vi "LoadDeviceList.vi"(8 "error in":errorcluster, 9 "usb/RS170":bool, 11 "path to XML document":path) -> (0 "error out":errorcluster, 1 "parse errors":string, 3 "DeviceList":T2(array[cluster]) {"Acquisition Parameters"."White level" scale=0.3..1.26 scale format="%#_2f"; "Acquisition Parameters"."Saturation" scale=0.5..1.5 scale format="%#_3f"; "Acquisition Parameters"."Contrast" scale=0.4..1.5 scale format="%#_3f"; "Acquisition Parameters"."Brightness" scale=-50.0..50.0 scale format="%#_2f"; "Correction Parameters"."Movement Type" items=["Step", "Proportionnal"]; "Target"."X Target" format="%#_5g"; "Target"."Y Target" format="%#_5g"; "Detection Parameters"."Max Intensity%" max=100 step=1})   [LabVIEW 2013]
uses:
  <vilib>/xml/Load XML File.vi
  <vilib>/xml/NI_XML.lvlib
  <resource>/objmgr/DOMUserDefRef.rc
panel:
  out "ImageServer":cluster{"IPAddress":string, "Port":i32}
  out "YCalibration":cluster{dbl, dbl}[](graph)
  out "XCalibration":cluster{dbl, dbl}[](graph)
  out "ID":i32
  out "Name":string
  out "DeviceID":T1
  out "Reference Path":path
  out "Background Path":path
  out "Acquisition Parameters":T3={"Brightness"=0.0, "Contrast"=1.0, "Saturation"=1.0, "White level"=0.7} {"White level" scale=0.3..1.26 scale format="%#_2f"; "Saturation" scale=0.5..1.5 scale format="%#_3f"; "Contrast" scale=0.4..1.5 scale format="%#_3f"; "Brightness" scale=-50.0..50.0 scale format="%#_2f"}
  out "Reverse":cluster{"Reverse X":bool, "Reverse Y":bool}
  out "Target":cluster{"X Target":sgl, "Y Target":sgl} {"X Target" format="%#_5g"; "Y Target" format="%#_5g"}
  out "Region of Interest":i32[](array[numeric])=[-1, -1, 32000, 32000]
  out "Correction Parameters":cluster{"X":sgl, "Y":sgl, "Movement Type":u16}={"X"=5.0, "Y"=5.0, "Movement Type"=0} {"Movement Type" items=["Step", "Proportionnal"]}
  out "Detection Parameters":T4 {"Max Intensity%" max=100 step=1}
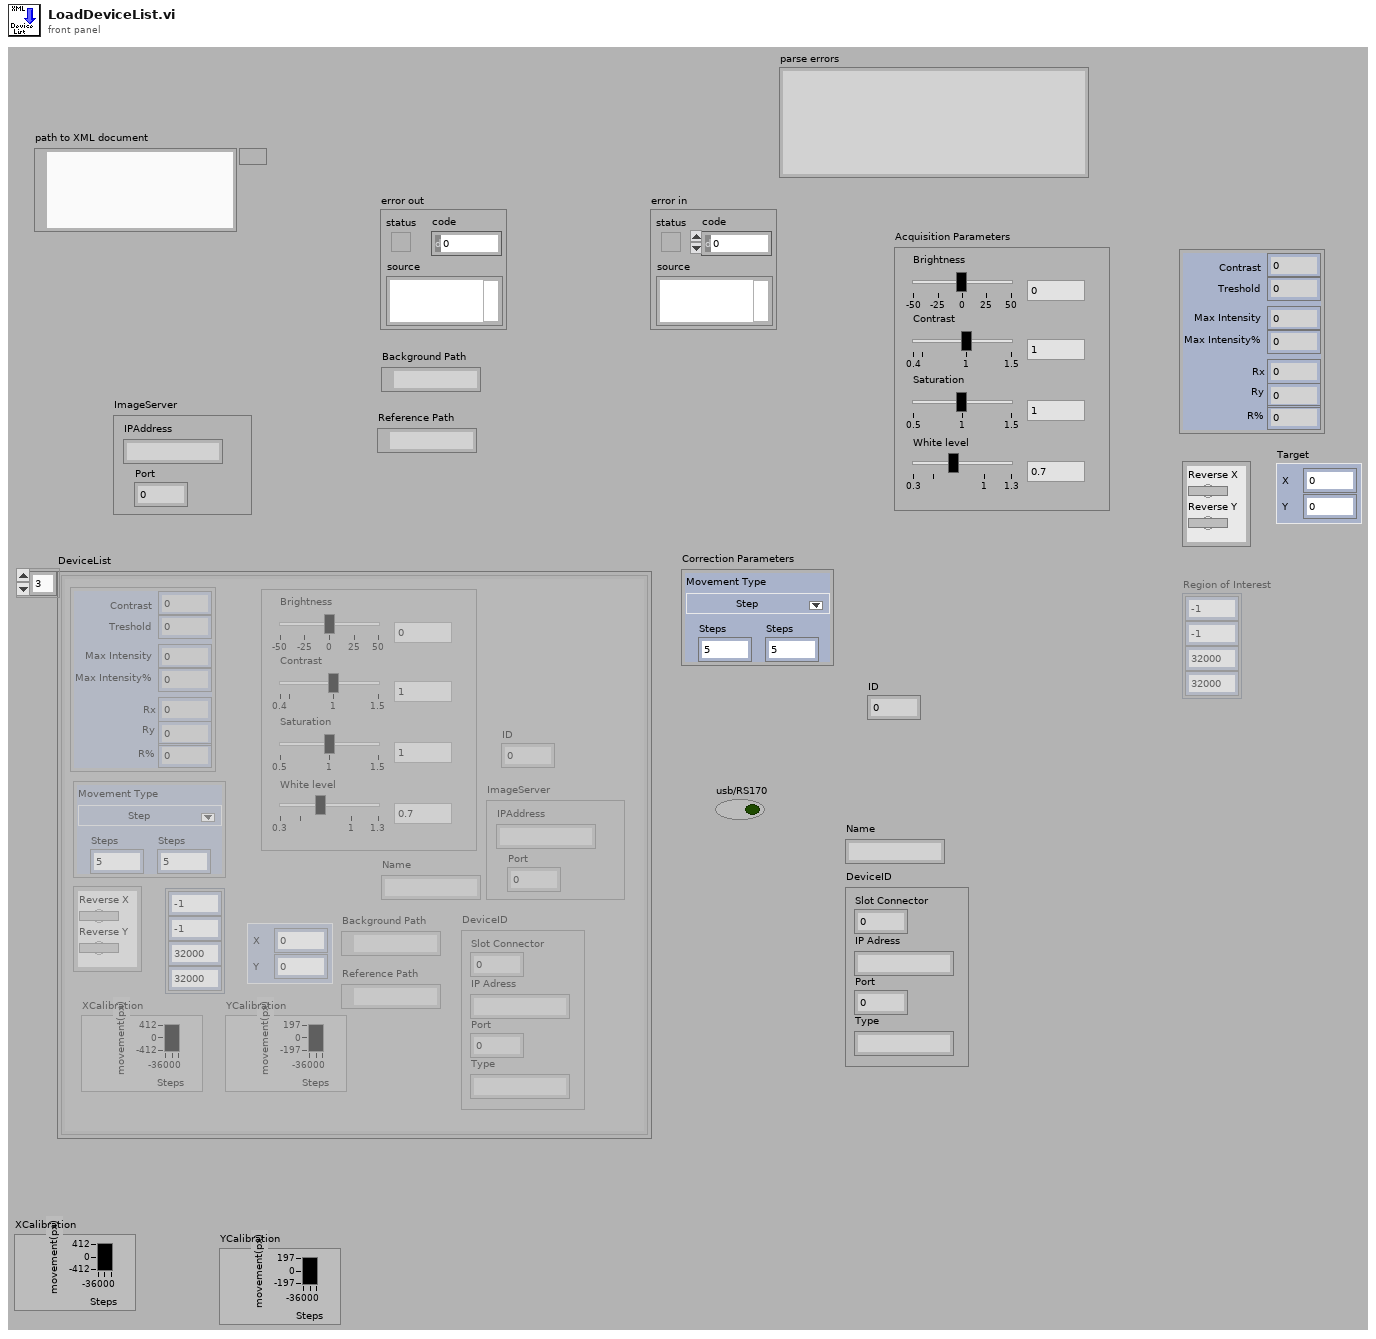
[diagram p1: front panel]
types:
  T1 = cluster{"Slot Connector":i32, "IP Adress":string, "Port":i32, "Type":string}
  T2 = cluster{"ID":dbl, "Name":string, "DeviceID":cluster{"Slot Connector":i32, "IP Adress":string, "Port":i32, "Type":string}, "Detection Parameters":cluster{"Contrast":i32, "Treshold":u8, "Max Intensity":i32, "Max Intensity%":u8, "Rx":i32, "Ry":i32, "R%":sgl}, "Reverse":cluster{"Reverse X":bool, "Reverse Y":bool}, "Target":cluster{"X Target":sgl, "Y Target":sgl}, "Region of Interest":i32[], "Correction Parameters":cluster{"X":sgl, "Y":sgl, "Movement Type":u16}, "Acquisition Parameters":cluster{"Brightness":dbl, "Contrast":dbl, "Saturation":dbl, "White level":dbl}, "Background Path":path, "Reference Path":path, "XCalibration":cluster{dbl, dbl}[], "YCalibration":cluster{dbl, dbl}[], "ImageServer":cluster{"IPAddress":string, "Port":i32}}[]
  T3 = cluster{"Brightness":dbl, "Contrast":dbl, "Saturation":dbl, "White level":dbl}
  T4 = cluster{"Contrast":i32, "Treshold":u8, "Max Intensity":i32, "Max Intensity%":u8, "Rx":i32, "Ry":i32, "R%":sgl}
  T5 = cluster{"Slot Connector":i32, "Name":string, "DeviceID":cluster{"Slot Connector":i32, "IP Adress":string, "Port":i32, "Type":string}, "Detection Parameters":cluster{"Contrast":i32, "Treshold":i32, "Max Intensity":i32, "Max Intensity%":i32, "Rx":i32, "Ry":i32, "R%":i32}, "Reverse":cluster{"Reverse X":bool, "Reverse Y":bool}, "Target":cluster{"X Target":sgl, "Y Target":sgl}, "Region of Interest":i32[], "Correction Parameters":cluster{"X":i32, "Y":i32, "Movement Type":u16}, "Acquisition Parameters":cluster{"Brightness":dbl, "Contrast":dbl, "Saturation":dbl, "White level":dbl}, "Background Path":path, "Reference Path":path, "XCalibration":cluster{dbl, dbl}[], "XCalibration 2":cluster{dbl, dbl}[], "ImageServer":cluster{"IPAddress":string, "Port":i32}}
  T6 = cluster{"Contrast":i32, "Name":string, "DeviceID":cluster{"Slot Connector":i32, "IP Adress":string, "Port":i32, "Type":string}, "Detection Parameters":cluster{"Contrast":i32, "Treshold":i32, "Max Intensity":i32, "Max Intensity%":i32, "Rx":i32, "Ry":i32, "R%":i32}, "Reverse":cluster{"Reverse X":bool, "Reverse Y":bool}, "Target":cluster{"X Target":sgl, "Y Target":sgl}, "Region of Interest":i32[], "Correction Parameters":cluster{"X":i32, "Y":i32, "Movement Type":u16}, "Acquisition Parameters":cluster{"Brightness":dbl, "Contrast":dbl, "Saturation":dbl, "White level":dbl}, "Background Path":path, "Reference Path":path, "XCalibration":cluster{dbl, dbl}[], "YCalibration":cluster{dbl, dbl}[], "ImageServer":cluster{"IPAddress":string, "Port":i32}}
  T7 = cluster{"Contrast":i32, "Name":string, "DeviceID":cluster{"Slot Connector":i32, "IP Adress":string, "Port":i32, "Type":string}, "Detection Parameters":cluster{"Contrast":i32, "Treshold":i32, "Max Intensity":i32, "Max Intensity%":i32, "Rx":i32, "Ry":i32, "R%":i32}, "Reverse":cluster{"Reverse X":bool, "Reverse Y":bool}, "Target":cluster{"X Target":sgl, "Y Target":sgl}, "Region of Interest":i32[], "Correction Parameters":cluster{"X":i32, "Y":i32, "Movement Type":u16}, "Acquisition Parameters":cluster{"Brightness":dbl, "Contrast":dbl, "Saturation":dbl, "White level":dbl}, "Background Path":path, "Reference Path":path, "XCalibration":cluster{dbl, dbl}[], "YCalibration":cluster{dbl, dbl}[], "ImageServer":cluster{"IPAddress":string, "Port":i32}}[]
  T8 = cluster{"ID":i32, "Name":string, "DeviceID":cluster{"Slot Connector":i32, "IP Adress":string, "Port":i32, "Type":string}, "Detection Parameters":cluster{"Contrast":i32, "Treshold":u8, "Max Intensity":i32, "Max Intensity%":u8, "Rx":i32, "Ry":i32, "R%":sgl}, "Reverse":cluster{"Reverse X":bool, "Reverse Y":bool}, "Target":cluster{"X Target":sgl, "Y Target":sgl}, "Region of Interest":i32[], "Correction Parameters":cluster{"X":sgl, "Y":sgl, "Movement Type":u16}, "Acquisition Parameters":cluster{"Brightness":dbl, "Contrast":dbl, "Saturation":dbl, "White level":dbl}, "Background Path":path, "Reference Path":path, "XCalibration":cluster{dbl, dbl}[], "YCalibration":cluster{dbl, dbl}[], "ImageServer":cluster{"IPAddress":string, "Port":i32}}
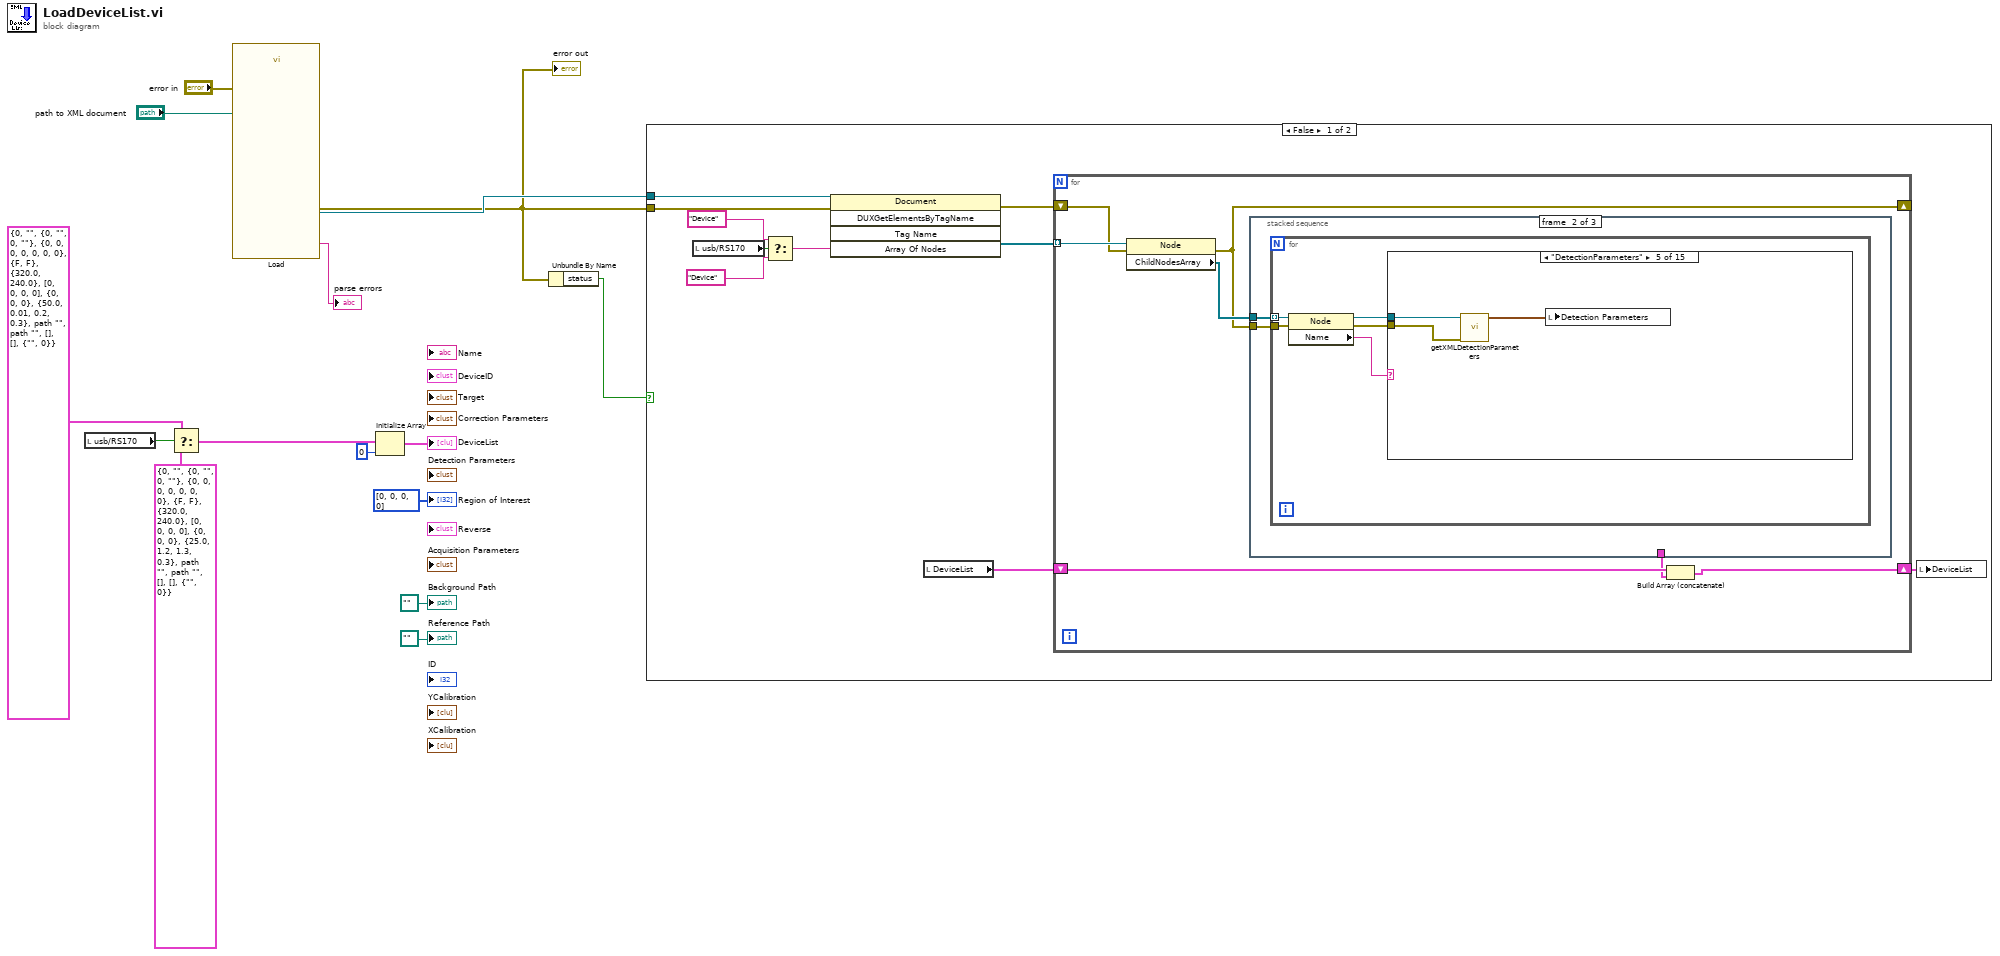
[diagram p0: block diagram]
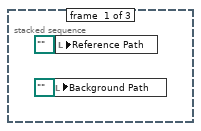
[diagram p2: hidden frame]
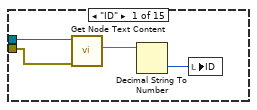
[diagram p3: hidden frame]
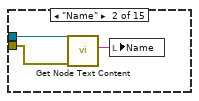
[diagram p4: hidden frame]
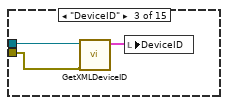
[diagram p5: hidden frame]
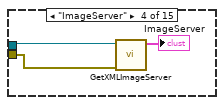
[diagram p6: hidden frame]
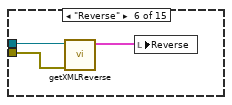
[diagram p7: hidden frame]
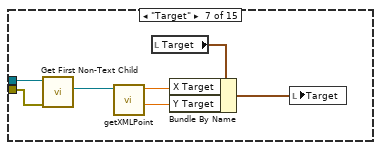
[diagram p8: hidden frame]
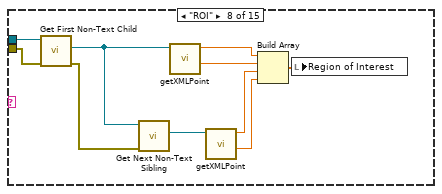
[diagram p9: hidden frame]
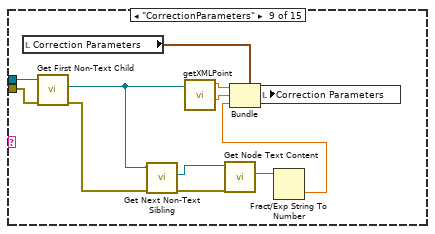
[diagram p10: hidden frame]
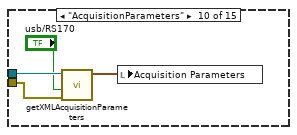
[diagram p11: hidden frame]
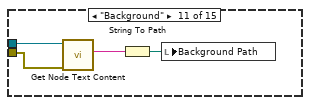
[diagram p12: hidden frame]
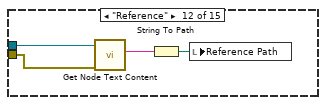
[diagram p13: hidden frame]
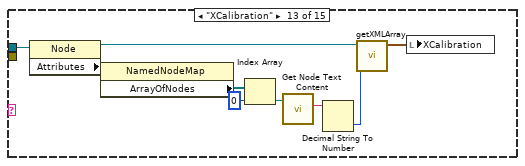
[diagram p14: hidden frame]
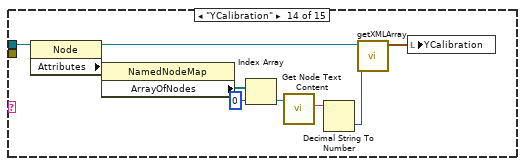
[diagram p15: hidden frame]
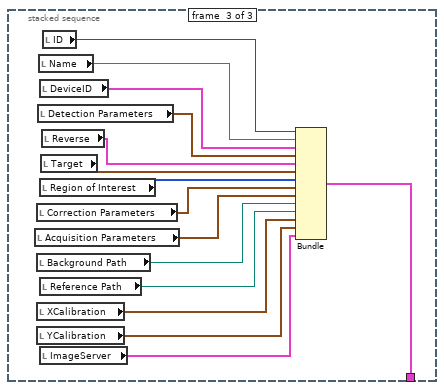
[diagram p17: hidden frame]
diagram:
  n1 = local read "usb/RS170"() -> (w6:bool)
  n2 = Select(t=T5 {"Slot Connector"=0, "Name"="", "DeviceID"={"Slot Connector"=0, "IP Adress"="", "Port"=0, "Type"=""}, "Detection Parameters"={"Contrast"=0, "Treshold"=0, "Max Intensity"=0, "Max Intensity%"=0, "Rx"=0, "Ry"=0, "R%"=0}, "Reverse"={"Reverse X"=FALSE, "Reverse Y"=FALSE}, "Target"={"X Target"=320.0, "Y Target"=240.0}, "Region of Interest"=[0, 0, 0, 0], "Correction Parameters"={"X"=0, "Y"=0, "Movement Type"=0}, "Acquisition Parameters"={"Brightness"=50.0, "Contrast"=0.01, "Saturation"=0.2, "White level"=0.3}, "Background Path"=path "", "Reference Path"=path "", "XCalibration"=[], "XCalibration 2"=[], "ImageServer"={"IPAddress"="", "Port"=0}} ("Cluster"), s=w6, f=T6 {"Contrast"=0, "Name"="", "DeviceID"={"Slot Connector"=0, "IP Adress"="", "Port"=0, "Type"=""}, "Detection Parameters"={"Contrast"=0, "Treshold"=0, "Max Intensity"=0, "Max Intensity%"=0, "Rx"=0, "Ry"=0, "R%"=0}, "Reverse"={"Reverse X"=FALSE, "Reverse Y"=FALSE}, "Target"={"X Target"=320.0, "Y Target"=240.0}, "Region of Interest"=[0, 0, 0, 0], "Correction Parameters"={"X"=0, "Y"=0, "Movement Type"=0}, "Acquisition Parameters"={"Brightness"=25.0, "Contrast"=1.2, "Saturation"=1.3, "White level"=0.3}, "Background Path"=path "", "Reference Path"=path "", "XCalibration"=[], "YCalibration"=[], "ImageServer"={"IPAddress"="", "Port"=0}} ("Cluster")) -> (s? t:f=w3:T6)
  n3 = call-poly <vilib>:"Load.vi"("path to XML document"="path to XML document", "error in (no error)"="error in") -> ("DOM document out"=w13:refnum<k20>, "parse errors"=→"parse errors":string, "error out"=w9:errorcluster)  [unwired: 11 in]
  "error out" <- w9
  n4 = Initialize Array(w3, 0 ("dimension size")) -> (→"DeviceList":T7)
  n5 = Unbundle By Name(w9) -> ("status"=w10:bool)
  n6 = case shown="False" w10 {
    tunnel: w13 -> [w25 _]
    tunnel: w9 -> [w24 _]
    frame False {
      n7 = local read "usb/RS170"() -> (w18:bool)
      n8 = Select(t="Device" ("Tag Name"), s=w18, f="Device" ("Tag Name")) -> (s? t:f=w16:string)
      n9 = invoke class="Document" method="DUXGetElementsByTagName"(reference=w25, error in=w24, "Tag Name"=w16) -> (error out=w22:errorcluster, "Array Of Nodes"=w23:refnum<k20>[])  [unwired: 2 in, 3 out]
      n10 = local read "DeviceList"() -> (w21:T2)
      n11 = for {
        tunnel: w23 -> [w32] mode=indexing
        shift-right: [w29] -> _
        shift-left: w22 -> [w31]
        shift-right: [w27] -> w20
        shift-left: w21 -> [w28]
        n12 = property class="Node"(reference=w32, error in=w31) -> (error out=w29:errorcluster, "ChildNodesArray"=w30:refnum<k20>[])  [unwired: 1 out]
        n13 = stacked-sequence {
          tunnel: w30 -> [_ w36 _]
          tunnel: w29 -> [_ w35 _]
          tunnel: [_ _ w134] -> w26
          frame #0 {
            n14 = local write "Background Path"(path "" ("Background Path")) -> ()
            n15 = local write "Reference Path"(path "" ("Reference Path")) -> ()
          }
          frame #1 {
            n16 = for {
              tunnel: w36 -> [w41] mode=indexing
              tunnel: w35 -> [w39]
              n17 = property class="Node"(reference=w41, error in=w39) -> (reference out=w40:refnum<k20>, error out=w38:errorcluster, "Name"=w37:string)
              n18 = case shown="\"DetectionParameters\"" w37 {
                tunnel: w40 -> [w45 w47 w51 w54 w57 w60 w65 w72 w83 w93 w97 w101 w110 w111 _]
                tunnel: w38 -> [w44 w46 w50 w53 w56 w59 w64 w69 w82 w92 w96 w100 _ _ _]
                frame "ID" {
                  n19 = call <vilib>:"Get Node Text Content.vi"("error in (no error)"=w44, "node in"=w45) -> ("node text"=w43:string)  [unwired: 7 in, 2 out]
                  n20 = Decimal String To Number(string=w43) -> (number=w42:i32)  [unwired: 2 in, 1 out]
                  n21 = local write "ID"(w42) -> ()
                }
                frame "Name" {
                  n22 = call <vilib>:"Get Node Text Content.vi"("error in (no error)"=w46, "node in"=w47) -> ("node text"=w48:string)  [unwired: 7 in, 2 out]
                  n23 = local write "Name"(w48) -> ()
                }
                frame "DeviceID" {
                  n24 = call "GetXMLDeviceID.vi"("error in"=w50, "Node"=w51) -> ("DeviceID"=w49:T1)  [unwired: 8 in, 1 out]
                  n25 = local write "DeviceID"(w49) -> ()
                }
                frame "ImageServer" {
                  n26 = call "GetXMLImageServer.vi"("error in"=w53, "Node"=w54) -> ("ImageServer"=→"ImageServer":cluster{"IPAddress":string, "Port":i32})  [unwired: 8 in, 1 out]
                }
                frame "DetectionParameters" {
                  n27 = call "getXMLDetectionParameters.vi"("error in"=w56, "Detection Parameters Node"=w57) -> ("Detection Parameters"=w55:T4)  [unwired: 7 in, 1 out]
                  n28 = local write "Detection Parameters"(w55) -> ()
                }
                frame "Reverse" {
                  n29 = call "getXMLReverse.vi"("error in"=w59, "Node"=w60) -> ("Reverse"=w58:cluster{"Reverse X":bool, "Reverse Y":bool})  [unwired: 8 in, 1 out]
                  n30 = local write "Reverse"(w58) -> ()
                }
                frame "Target" {
                  n31 = call <vilib>:"Get First Non-Text Child.vi"("error in (no error)"=w64, "node in"=w65) -> ("child node"=w63:refnum<k20>)  [unwired: 6 in, 3 out]
                  n32 = call "getXMLPoint.vi"("Point Node"=w63) -> ("y"=w66:dbl, "x"=w67:dbl)  [unwired: 9 in]
                  n33 = local read "Target"() -> (w61:cluster{"X Target":sgl, "Y Target":sgl})
                  n34 = Bundle By Name(cluster=w61, "X Target"=w67, "Y Target"=w66) -> (w62:cluster{"X Target":sgl, "Y Target":sgl})
                  n35 = local write "Target"(w62) -> ()
                }
                frame "ROI" {
                  n36 = call <vilib>:"Get First Non-Text Child.vi"("error in (no error)"=w69, "node in"=w72) -> ("error out"=w71:errorcluster, "child node"=w68:refnum<k20>)  [unwired: 6 in, 2 out]
                  n37 = call <vilib>:"Get Next Non-Text Sibling.vi"("error in (no error)"=w71, "node in"=w68) -> ("sibling node"=w70:refnum<k20>)  [unwired: 6 in, 3 out]
                  n38 = call "getXMLPoint.vi"("Point Node"=w68) -> ("y"=w75:dbl, "x"=w76:dbl)  [unwired: 9 in]
                  n39 = call "getXMLPoint.vi"("Point Node"=w70) -> ("y"=w74:dbl, "x"=w73:dbl)  [unwired: 9 in]
                  n40 = Build Array(w76, w75, w73, w74) -> (w77:dbl[])
                  n41 = local write "Region of Interest"(w77) -> ()
                }
                frame "CorrectionParameters" {
                  n42 = local read "Correction Parameters"() -> (w88:cluster{"X":sgl, "Y":sgl, "Movement Type":u16})
                  n43 = call <vilib>:"Get First Non-Text Child.vi"("error in (no error)"=w82, "node in"=w83) -> ("error out"=w80:errorcluster, "child node"=w81:refnum<k20>)  [unwired: 6 in, 2 out]
                  n44 = call <vilib>:"Get Next Non-Text Sibling.vi"("error in (no error)"=w80, "node in"=w81) -> ("error out"=w78:errorcluster, "sibling node"=w79:refnum<k20>)  [unwired: 6 in, 2 out]
                  n45 = call "getXMLPoint.vi"("Point Node"=w81) -> ("y"=w86:dbl, "x"=w87:dbl)  [unwired: 9 in]
                  n46 = call <vilib>:"Get Node Text Content.vi"("error in (no error)"=w78, "node in"=w79) -> ("node text"=w89:string)  [unwired: 7 in, 2 out]
                  n47 = Fract/Exp String To Number(string=w89) -> (number=w85:dbl)  [unwired: 3 in, 1 out]
                  n48 = Bundle(cluster=w88, "X"=w87, "Y"=w86, "Movement Type"=w85) -> (w84:cluster{"X":sgl, "Y":sgl, "Movement Type":u16})
                  n49 = local write "Correction Parameters"(w84) -> ()
                }
                frame "AcquisitionParameters" {
                  n50 = call "getXMLAcquisitionParameters.vi"("error in"=w92, "usb/RS170"="usb/RS170", "Axquisition Parameters Node"=w93) -> ("Acquisition Parameters"=w91:T3)  [unwired: 7 in, 1 out]
                  n51 = local write "Acquisition Parameters"(w91) -> ()
                }
                frame "Background" {
                  n52 = call <vilib>:"Get Node Text Content.vi"("error in (no error)"=w96, "node in"=w97) -> ("node text"=w95:string)  [unwired: 7 in, 2 out]
                  n53 = String To Path(string=w95) -> (path=w94:path)
                  n54 = local write "Background Path"(w94) -> ()
                }
                frame "Reference" {
                  n55 = call <vilib>:"Get Node Text Content.vi"("error in (no error)"=w100, "node in"=w101) -> ("node text"=w99:string)  [unwired: 7 in, 2 out]
                  n56 = String To Path(string=w99) -> (path=w98:path)
                  n57 = local write "Reference Path"(w98) -> ()
                }
                frame "XCalibration" {
                  n58 = property class="Node"(reference=w110) -> (reference out=w104:refnum<k20>, "Attributes"=w109:refnum<k20>)  [unwired: 1 in, 1 out]
                  n59 = property class="NamedNodeMap"(reference=w109) -> ("ArrayOfNodes"=w108:refnum<k20>[])  [unwired: 1 in, 2 out]
                  n60 = Index Array(array=w108, index=0) -> (element=w106:refnum<k20>)
                  n61 = call <vilib>:"Get Node Text Content.vi"("node in"=w106) -> ("node text"=w105:string)  [unwired: 8 in, 2 out]
                  n62 = Decimal String To Number(string=w105) -> (number=w103:i32)  [unwired: 2 in, 1 out]
                  n63 = call "getXMLArray.vi"("size"=w103, "Array Node"=w104) -> ("Array"=w102:cluster{dbl, dbl}[])  [unwired: 9 in]
                  n64 = local write "XCalibration"(w102) -> ()
                }
                frame "YCalibration" {
                  n65 = property class="Node"(reference=w111) -> (reference out=w114:refnum<k20>, "Attributes"=w119:refnum<k20>)  [unwired: 1 in, 1 out]
                  n66 = property class="NamedNodeMap"(reference=w119) -> ("ArrayOfNodes"=w118:refnum<k20>[])  [unwired: 1 in, 2 out]
                  n67 = Index Array(array=w118, index=0) -> (element=w116:refnum<k20>)
                  n68 = call <vilib>:"Get Node Text Content.vi"("node in"=w116) -> ("node text"=w115:string)  [unwired: 8 in, 2 out]
                  n69 = Decimal String To Number(string=w115) -> (number=w113:i32)  [unwired: 2 in, 1 out]
                  n70 = call "getXMLArray.vi"("size"=w113, "Array Node"=w114) -> ("Array"=w112:cluster{dbl, dbl}[])  [unwired: 9 in]
                  n71 = local write "YCalibration"(w112) -> ()
                }
                frame Default {
                }
              }
            }
          }
          frame #2 {
            n72 = local read "Acquisition Parameters"() -> (w128:T3)
            n73 = local read "Correction Parameters"() -> (w129:cluster{"X":sgl, "Y":sgl, "Movement Type":u16})
            n74 = local read "Background Path"() -> (w127:path)
            n75 = local read "XCalibration"() -> (w122:cluster{dbl, dbl}[])
            n76 = local read "YCalibration"() -> (w121:cluster{dbl, dbl}[])
            n77 = local read "Detection Parameters"() -> (w133:T4)
            n78 = local read "Name"() -> (w124:string)
            n79 = local read "DeviceID"() -> (w125:T1)
            n80 = local read "Region of Interest"() -> (w130:i32[])
            n81 = local read "Reference Path"() -> (w126:path)
            n82 = local read "ImageServer"() -> (w120:cluster{"IPAddress":string, "Port":i32})
            n83 = local read "Target"() -> (w131:cluster{"X Target":sgl, "Y Target":sgl})
            n84 = local read "Reverse"() -> (w132:cluster{"Reverse X":bool, "Reverse Y":bool})
            n85 = local read "ID"() -> (w123:i32)
            n86 = Bundle("ID"=w123, "Name"=w124, "DeviceID"=w125, "Detection Parameters"=w133, "Reverse"=w132, "Target"=w131, "Region of Interest"=w130, "Correction Parameters"=w129, "Acquisition Parameters"=w128, "Background Path"=w127, "Reference Path"=w126, "XCalibration"=w122, "YCalibration"=w121, "ImageServer"=w120) -> (w134:T8)  [unwired: 1 in]
          }
        }
        n87 = Build Array (concatenate)(w28, w26) -> (w27:T2)
      }
      n88 = local write "DeviceList"(w20) -> ()
    }
    frame True {
    }
  }
  "Region of Interest" <- i32[] [0, 0, 0, 0] ("Region of Interest")
  "Background Path" <- path "" ("Background Path")
  "Reference Path" <- path "" ("Background Path")
